vi "GlobalCameraDebugTemperature.vi"() -> ()   [LabVIEW 2013]
panel:
  in  "Fast Slow Debug":enum32{"Normal", "Debug"}(radio)
  in  "temperature":i32=-70
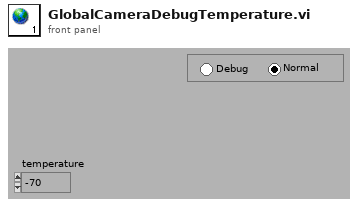
[diagram p1: front panel]
diagram:
